vi "Brutale_soluzione.vi"() -> ()   [LabVIEW 2016]
panel:
  in  "stop":bool
  in  "Remote host/IP address":string="84.253.163.35"
  out "http_address":string
  in  "password":string="gamma2018"
  in  "username":string="admin"
  in  "Stringa Comando":string="/cgi-bin/snapshot.cgi?"
  # "rtsp://admin:gamma2018@84.253.163.35:554/cam/realmonitor?channel=1&subtype=1"
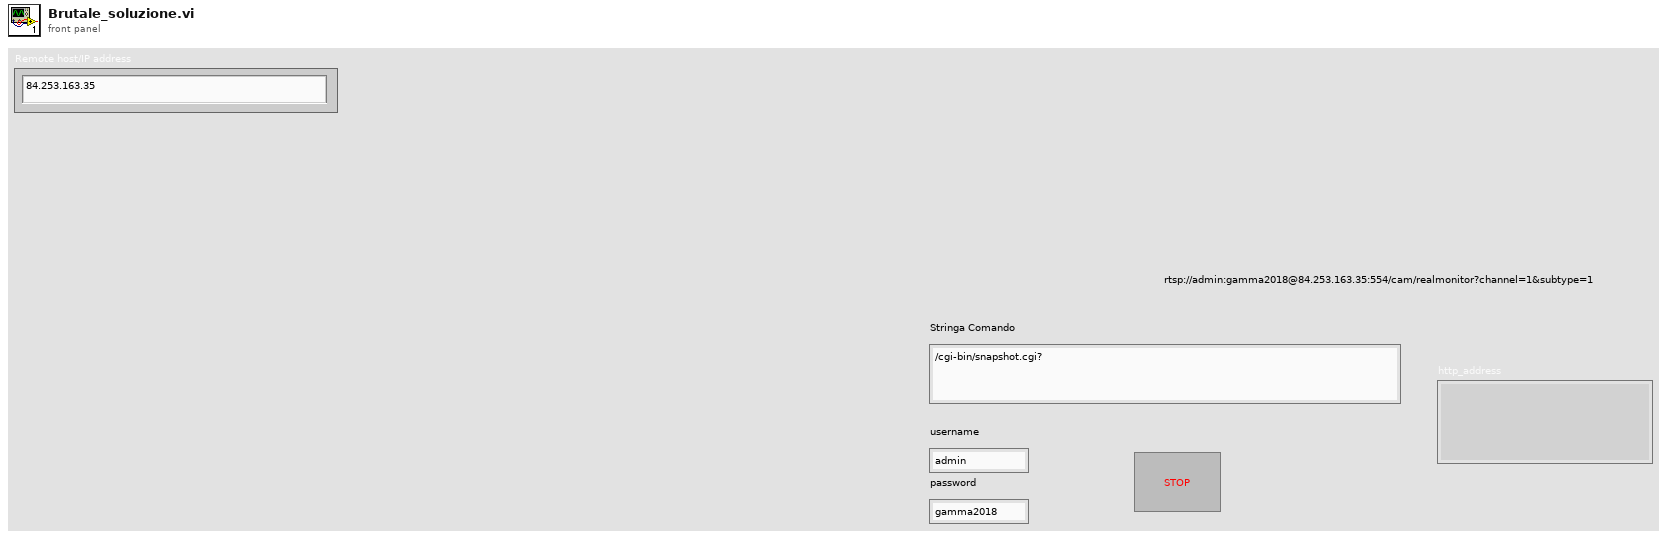
[diagram p1: front panel]
types:
  T1 = typedef "LabVIEWHTTPClient.lvlib/ClientHandle.ctl" = refnum<k1>
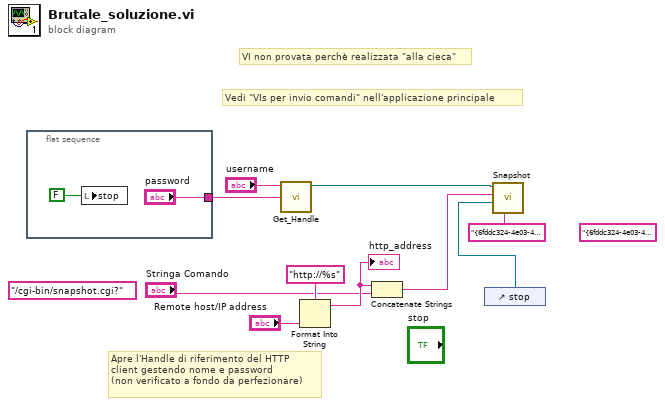
[diagram p0: block diagram]
diagram:
  (unwired) "{6fddc324-4e03-4bfe-b185-3d77768dc90e}" ("Dest Format")
  (unwired) "/cgi-bin/snapshot.cgi?" ("Stringa Comando")
  # "Apre l'Handle di riferimento del HTTP\nclient gestendo nome e password \n(non verificato a fondo da perfezionare)"
  # "VI non provata perchè realizzata \"alla cieca\""
  # "Vedi \"VIs per invio comandi\" nell'applicazione principale"
  n1 = flat-sequence {
    tunnel: ["password"] -> w6
    frame #0 {
      n2 = local write "stop"(FALSE) -> ()
    }
  }
  n3 = call "Get_Handle.vi"("password"=w6, "username"="username") -> ("Refnum out"=w5:T1)  [unwired: 9 in]
  n4 = Format Into String(format string="http://%s", "Remote host/IP address") -> (resulting string=w9:string)  [unwired: 2 in, 1 out]
  "http_address" <- w9
  n5 = Concatenate Strings(w9, "Stringa Comando") -> (w3:string)
  n6 = control-ref of="stop"() -> (w2:refnum<vi>)
  n7 = call "Snapshot.vi"("Dest Format"="{6fddc324-4e03-4bfe-b185-3d77768dc90e}", "Stop Ref"=w2, "Value"=w3, "Refnum in"=w5) -> ()  [unwired: 7 in, 1 out]
